vi "PH_BL-Master.set GUI Refs.vi"(0 "i ref in":refnum<vi>, 2 "Class":string, 3 "PH_BL-Master GUI Refs":T2, 4 "System Information GUI Refs":T1, 5 "error in":errorcluster) -> (14 "i ref out":refnum<vi>, 19 "error out":errorcluster)   [LabVIEW 2014, in "PH_BL-Master.lvlib"]
uses:
  PH_BL-Master.lvlib
  PH_BL-Master.GUI Refs.ctl
  PH_SystemInformation/PH_SystemInformation.GUI Refs.ctl
  PH_4_Pos_Selector/PH_4_Pos_Selector.Position Selector.ctl
  PH_StatusHandler/PH_StatusHandler.Status.ctl
  PH_SystemInformation/PH_SystemInformation.lvlib
  PH_4_Pos_Selector/PH_4_Pos_Selector.lvlib
  PH_StatusHandler/PH_StatusHandler.lvlib
panel:
  # "Attention Attention Attention Attention Attention Attention Attention Attention Attention \n\nAt own attributes (and within all relevant sub-VIs), the GUI references of\n\nboolean and numeric GUI elements MUST be of strict type def, while those of\npicture GUI elements NOT!\n\nAlso NOT: The references for the instances rings!\n\nOtherwise build will fail!!!"
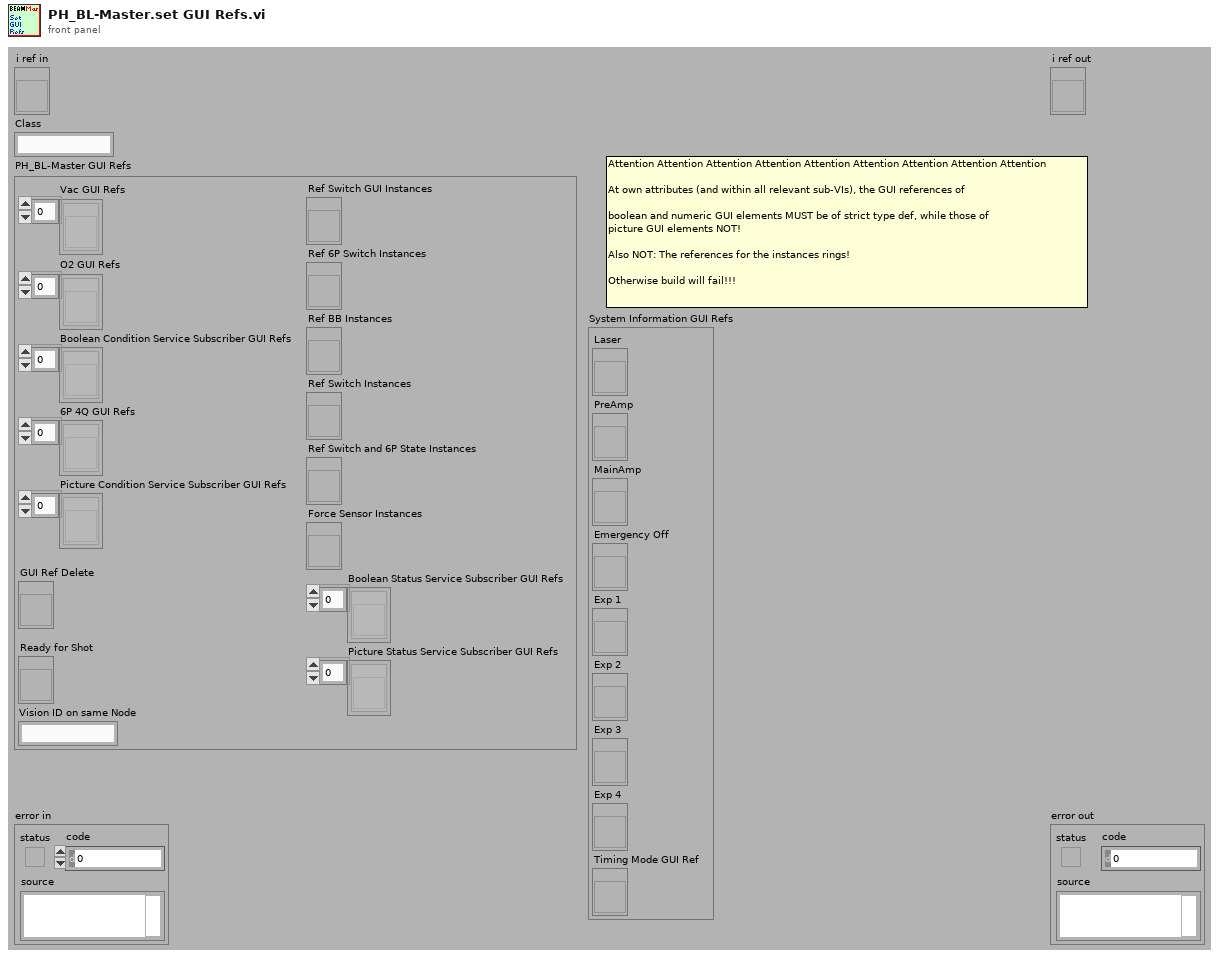
[diagram p1: front panel]
types:
  T1 = typedef "PH_SystemInformation.lvlib/PH_SystemInformation.GUI Refs.ctl" = cluster{"Laser":refnum<vi>, "PreAmp":refnum<vi>, "MainAmp":refnum<vi>, "Emergency Off":refnum<vi>, "Exp 1":refnum<vi>, "Exp 2":refnum<vi>, "Exp 3":refnum<vi>, "Exp 4":refnum<vi>, "Timing Mode GUI Ref":refnum<vi>}
  T2 = typedef "PH_BL-Master.lvlib/PH_BL-Master.GUI Refs.ctl" = cluster{"Vac GUI Refs":refnum<vi>[], "O2 GUI Refs":refnum<vi>[], "Ready for Shot":refnum<vi>, "Boolean Condition Service Subscriber GUI Refs":refnum<vi>[], "Vision ID on same Node":string, "Picture Condition Service Subscriber GUI Refs":refnum<vi>[], "6P 4Q GUI Refs":refnum<vi>[], "Ref Switch GUI Instances":refnum<vi>, "Ref 6P Switch Instances":refnum<vi>, "Ref BB Instances":refnum<vi>, "Ref Switch Instances":refnum<vi>, "Ref Switch and 6P State Instances":refnum<vi>, "Boolean Status Service Subscriber GUI Refs":refnum<vi>[], "Picture Status Service Subscriber GUI Refs":refnum<vi>[], "Force Sensor Instances":refnum<vi>, "GUI Ref Delete":refnum<vi>}
  T3 = typedef "PH_StatusHandler.lvlib/PH_StatusHandler.Status.ctl" = i16
  T4 = cluster{"GUI Ref":refnum<vi>, "Concentration":dbl, "State":T3}
  T5 = cluster{"GUI Ref":refnum<vi>, "Limit":dbl, "Curr Value":dbl, "in range":bool}
  T6 = typedef "PH_4_Pos_Selector.lvlib/PH_4_Pos_Selector.Position Selector.ctl" = u16
  T7 = cluster{"GUI Ref":refnum<vi>, "Selector":T6, "no Link?":bool}
  T8 = typedef "PH_BL-Master.lvlib/PH_BL-Master.i attribute.ctl" = cluster{"Remote controlled":bool, "Boolean Condition Service Subscriber":refnum<vi>[], "Picture Condition Service Subscriber":refnum<vi>[], "R2S":cluster{"GUI Ref":refnum<vi>, "State":bool}, "Vacua":cluster{"GUI Ref":refnum<vi>, "Limit":dbl, "Curr Value":dbl, "in range":bool}[], "O2 Inspection":cluster{"GUI Ref":refnum<vi>, "Concentration":dbl, "State":T3}[], "Boolean Status Service Subscriber":cluster{"GUI Ref":refnum<vi>, "Status":T3, "no Link?":bool, "Status Subscriber Class":T9}[], "Picture Status Service Subscriber":cluster{"GUI Ref":refnum<vi>, "Status":T3, "no Link?":bool, "Status Subscriber Class":T9}[], "6P 4Q Service Subscriber":cluster{"GUI Ref":refnum<vi>, "Selector":T6, "no Link?":bool}[], "Index of latest 6P 4Q changing Instance":i32, "Index of latest Picture Status changing Instance":i32, "Index of latest Boolean Status changing Instance":i32, "Vision ID on same Node":string, "Start Phase over?":bool, "GUI Ref Delete":refnum<vi>}
  T9 = typedef "PH_BL-Master.lvlib/PH_BL-Master.Status Subscriber Class.ctl" = enum16{"unknown", "Switch", "BB", "6P Switch", "Switch GUI", "Switch and 6P State", "Force Sensor"}
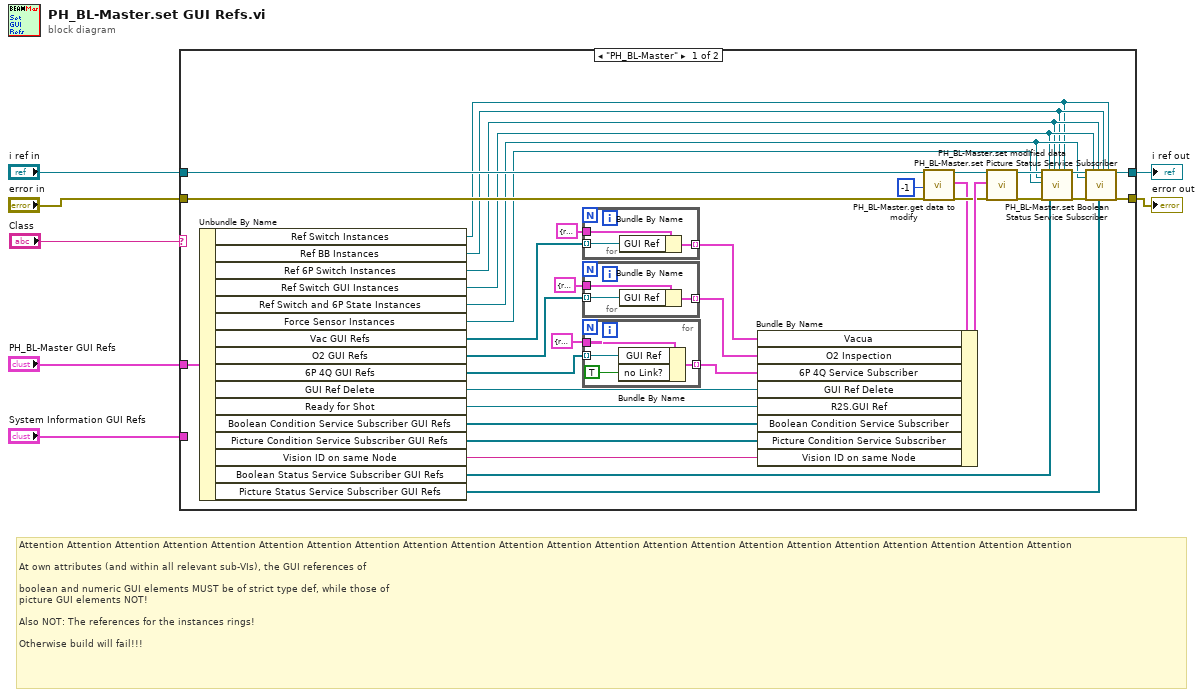
[diagram p0: block diagram]
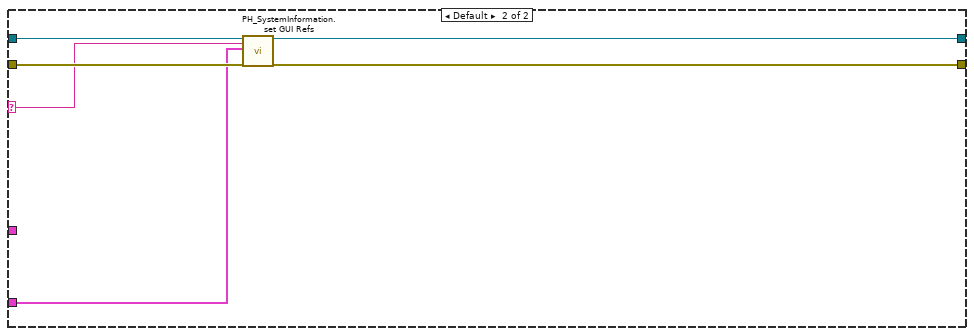
[diagram p2: hidden frame]
diagram:
  # "Attention Attention Attention Attention Attention Attention Attention Attention Attention Attention Attention Attention Attention Attention Attention Attention Attention Attention Attention Attention Attention Attention \n\nAt own attributes (and within all relevant sub-VIs), the GUI references of\n\nboolean and numeric GUI elements MUST be of strict type def, while those of\npicture GUI elements NOT!\n\nAlso NOT: The references for the instances rings!\n\nOtherwise build will fail!!!"
  n1 = case shown="\"PH_BL-Master\"" "Class" {
    selector: "Class" -> [_ w55]
    tunnel: [w12 w58] -> w7
    tunnel: "i ref in" -> [w40 w59]
    tunnel: [w11 w56] -> w5
    tunnel: "error in" -> [w38 w57]
    tunnel: "PH_BL-Master GUI Refs" -> [w30 _]
    tunnel: "System Information GUI Refs" -> [_ w54]
    frame "PH_BL-Master" {
      n2 = Unbundle By Name(w30) -> ("Ref Switch Instances"=w13:refnum<vi>, "Ref BB Instances"=w14:refnum<vi>, "Ref 6P Switch Instances"=w15:refnum<vi>, "Ref Switch GUI Instances"=w16:refnum<vi>, "Ref Switch and 6P State Instances"=w17:refnum<vi>, "Force Sensor Instances"=w10:refnum<vi>, "Vac GUI Refs"=w29:refnum<vi>[], "O2 GUI Refs"=w28:refnum<vi>[], "6P 4Q GUI Refs"=w27:refnum<vi>[], "GUI Ref Delete"=w26:refnum<vi>, "Ready for Shot"=w8:refnum<vi>, "Boolean Condition Service Subscriber GUI Refs"=w9:refnum<vi>[], "Picture Condition Service Subscriber GUI Refs"=w25:refnum<vi>[], "Vision ID on same Node"=w24:string, "Boolean Status Service Subscriber GUI Refs"=w18:refnum<vi>[], "Picture Status Service Subscriber GUI Refs"=w19:refnum<vi>[])
      n3 = for {
        tunnel: T5 {"GUI Ref"=refnum, "Limit"=0.0, "Curr Value"=0.0, "in range"=FALSE} ("Vacuum Dummy") -> [w53]
        tunnel: [w52] -> w32 mode=indexing
        tunnel: w29 -> [w51] mode=indexing
        n4 = Bundle By Name(cluster=w53, "GUI Ref"=w51) -> (w52:T5)
      }
      n5 = for {
        tunnel: T4 {"GUI Ref"=refnum, "Concentration"=0.0, "State"=0} ("O2 Information Dummy") -> [w50]
        tunnel: [w49] -> w31 mode=indexing
        tunnel: w28 -> [w48] mode=indexing
        n6 = Bundle By Name(cluster=w50, "GUI Ref"=w48) -> (w49:T4)
      }
      n7 = for {
        tunnel: [w47] -> w33 mode=indexing
        tunnel: T7 {"GUI Ref"=refnum, "Selector"=0, "no Link?"=FALSE} ("6P 4Q Service Subscriber") -> [w46]
        tunnel: w27 -> [w45] mode=indexing
        n8 = Bundle By Name(cluster=w46, "GUI Ref"=w45, "no Link?"=TRUE) -> (w47:T7)
      }
      n9 = call "PH_BL-Master.get data to modify.vi"("i ref in"=w40, "ms timeout (10000)"=-1, "error in (no error)"=w38) -> ("i ref out"=w41:refnum<vi>, "i attribute"=w37:T8, "error out"=w39:errorcluster)  [unwired: 13 in, 1 out]
      n10 = Bundle By Name(cluster=w37, "Vacua"=w32, "O2 Inspection"=w31, "6P 4Q Service Subscriber"=w33, "GUI Ref Delete"=w26, "R2S.GUI Ref"=w8, "Boolean Condition Service Subscriber"=w9, "Picture Condition Service Subscriber"=w25, "Vision ID on same Node"=w24) -> (w42:T8)
      n11 = call "PH_BL-Master.set modified data.vi"("i ref in"=w41, "i attribute"=w42, "error in (no error)"=w39) -> ("i ref out"=w20:refnum<vi>, "error out"=w22:errorcluster)  [unwired: 15 in]
      n12 = call "PH_BL-Master.set Boolean Status Service Subscriber.vi"("i ref in"=w20, "Ref Switch and 6P State Instances"=w17, "Force Sensor Instances"=w10, "error in"=w22, "Ref Switch GUI Instances"=w16, "Boolean Status Service Subscriber GUI Refs"=w18, "Ref 6P Switch Instances"=w15, "Ref BB Instances"=w14, "Ref Switch Instances"=w13) -> ("i ref out"=w21:refnum<vi>, "error out"=w23:errorcluster)  [unwired: 9 in]
      n13 = call "PH_BL-Master.set Picture Status Service Subscriber.vi"("i ref in"=w21, "Ref Switch and 6P State Instances"=w17, "error in"=w23, "Ref Switch GUI Instances"=w16, "Ref 6P Switch Instances"=w15, "Picture Status Service Subscriber GUI Refs"=w19, "Ref BB Instances"=w14, "Ref Switch Instances"=w13) -> ("i ref out"=w12:refnum<vi>, "error out"=w11:errorcluster)  [unwired: 10 in]
    }
    frame Default {
      n14 = call "PH_SystemInformation.set GUI Refs.vi"("i ref in"=w59, "Class"=w55, "System Information GUI Refs"=w54, "error in (no error)"=w57) -> ("i ref out"=w58:refnum<vi>, "error out"=w56:errorcluster)  [unwired: 14 in]
    }
  }
  "i ref out" <- w7
  "error out" <- w5
